vi "Get Data.vi"(8 "error in":errorcluster, 11 "PPT in":refnum<class "PPT.lvclass">) -> (0 "error out":errorcluster, 2 "DataOut":refnum<class "Data.lvclass">, 3 "PPT out":refnum<class "PPT.lvclass">)   [LabVIEW 2014, in "PPT Library.lvlib" / "PPT.lvclass"]
doc: "Retrieve the two PPT data products, pressure and temperature, and stuff them in a data object. Data will be retrieved for every object in the network."
uses:
  PPT.lvclass
  reusable/Data/Data.lvclass
  Data/PPT Data.lvclass
  Configurable Device/Configurable Device.lvclass/Configurable Device.ctl
  Data/PPT Data.lvclass/PPT Data.ctl
  reusable/Data/Data.lvclass/Data.ctl
  Configurable Device/Read ID.vi
  Data/Write T.vi
  Data/Write P.vi
  reusable/Data/Write Data ID.vi
  reusable/Data/Write measTime.vi
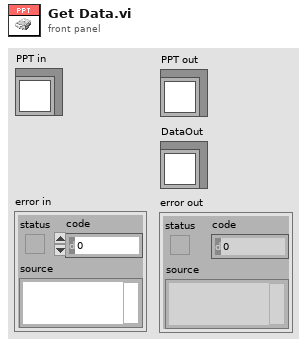
[diagram p1: front panel]
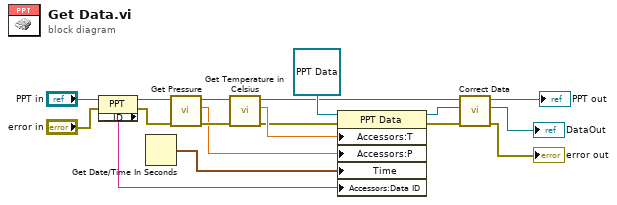
[diagram p0: block diagram]
diagram:
  n1 = property class="PPT"(reference="PPT in", error in="error in") -> (reference out=w11:refnum<class "PPT.lvclass">, error out=w9:errorcluster, "Accessors:ID"=w8:string)
  n2 = Get Date/Time In Seconds() -> (seconds since 1Jan1904=w17:timestamp)
  n3 = call "Get Pressure.vi"("error in"=w9, "PPT in"=w11) -> ("error out"=w15:errorcluster, "Pressure"=w14:dbl, "PPT out"=w16:refnum<class "PPT.lvclass">)  [unwired: 7 in]
  n4 = call "Get Temperature in Celsius.vi"("error in"=w15, "PPT in"=w16) -> ("error out"=w7:errorcluster, "Temperature"=w13:dbl, "PPT out"=w5:refnum<class "PPT.lvclass">)  [unwired: 7 in]
  n5 = property class="PPT Data"(reference=refnum<class "PPT Data.lvclass"> refnum ("PPT Data"), error in=w7, "Accessors:T"=w13, "Accessors:P"=w14, "Time"=w17, "Accessors:Data ID"=w8) -> (reference out=w6:refnum<class "PPT Data.lvclass">, error out=w4:errorcluster)
  n6 = call-dynamic "Correct Data.vi"("error in (no error)"=w4, "Data In"=w6, "PPT in"=w5) -> ("error out"=→"error out":errorcluster, "Data Out"=→"DataOut":refnum<class "Data.lvclass">, "PPT out"=→"PPT out":refnum<class "PPT.lvclass">)  [unwired: 6 in]
